vi "Check_UI2R_Validity.vi"(8 "error in (no error)":errorcluster, 9 "ControlValueUpdates[] in":T1[](array[typedef]), 10 "UI Filepath in":path, 11 "UI_Interaction_Manager in":refnum<class "UI_Interaction_Manager.lvclass">) -> (0 "error out":errorcluster, 1 "ControlValueUpdates[] out":T1[](array[typedef]), 2 "Valid?":bool, 3 "UI_Interaction_Manager out":refnum<class "UI_Interaction_Manager.lvclass">)   [LabVIEW 2011, in "UI_Interaction_Manager.lvclass"]
uses:
  UI_Interaction_Manager.lvclass
  TypeDefs/ControlValueUpdate.ctl
  UI_Interaction_Manager.lvclass/UI_Interaction_Manager.ctl
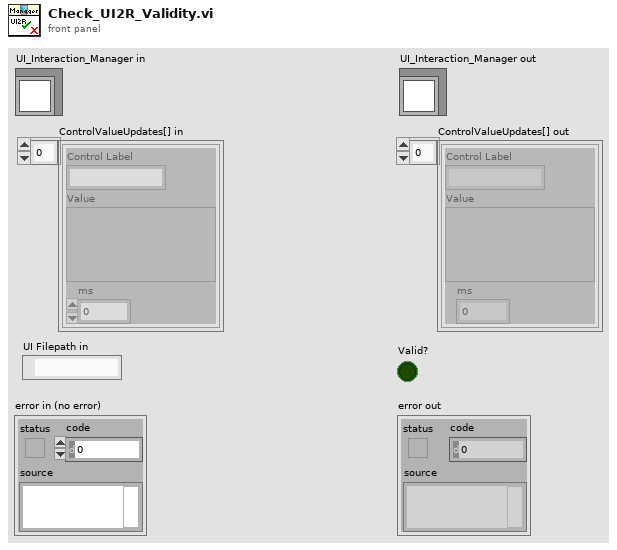
[diagram p1: front panel]
types:
  T1 = typedef "UI_Interaction_Manager.lvclass/ControlValueUpdate.ctl" = cluster{"Control Label":string, "Value":variant, "ms":u32}
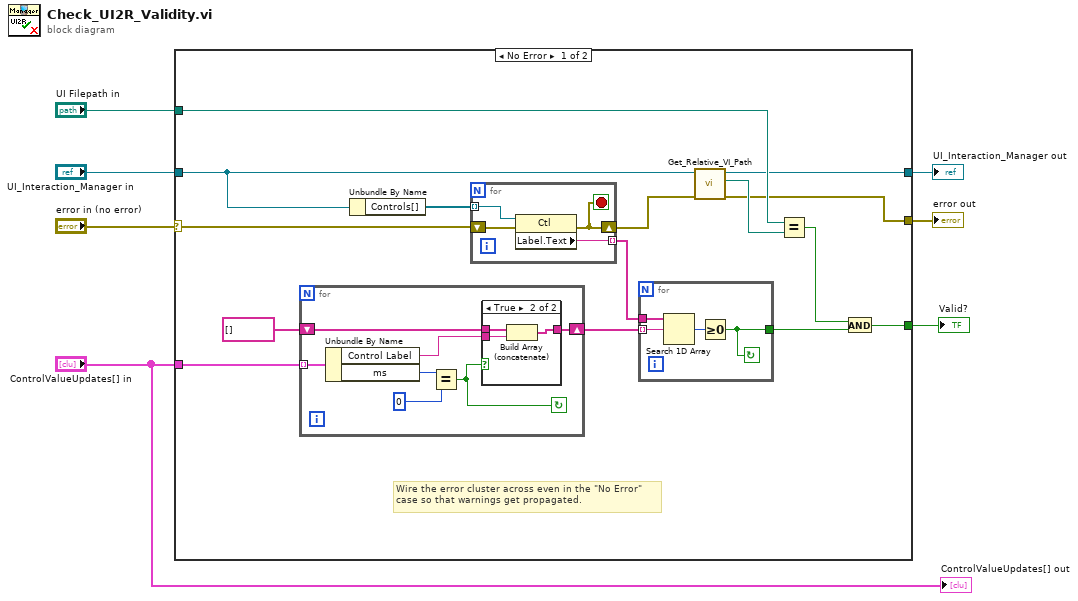
[diagram p0: block diagram]
diagram:
  n1 = case shown="No Error" "error in (no error)" {
    selector: "error in (no error)" -> [w16 w43]
    tunnel: [w11 w43] -> w6
    tunnel: [w12 w42] -> w4
    tunnel: "UI_Interaction_Manager in" -> [w17 w42]
    tunnel: "UI Filepath in" -> [w14 _]
    tunnel: "ControlValueUpdates[] in" -> [w22 _]
    tunnel: [w8 _] -> w1
    frame No Error {
      # "Wire the error cluster across even in the \"No Error\"\ncase so that warnings get propagated."
      n2 = for {
        tunnel: w22 -> [w37] mode=indexing
        shift-right: [w31] -> w19
        shift-left: string[] [] -> [w34]
        stop <- w33 continue-if-true
        n3 = Unbundle By Name(w37) -> ("Control Label"=w32:string, "ms"=w36:u32)
        n4 = Equal?(x=w36, y=u32 0) -> (x = y?=w33:bool)
        n5 = case shown="True" w33 {
          tunnel: w34 -> [w38 w41]
          tunnel: w32 -> [_ w40]
          tunnel: [w38 w39] -> w31
          frame False {
          }
          frame True {
            n6 = Build Array (concatenate)(w41, w40) -> (w39:string[])
          }
        }
      }
      n7 = Unbundle By Name(w17) -> ("Controls[]"=w20:refnum<vi>[])
      n8 = for {
        tunnel: w20 -> [w27] mode=indexing
        tunnel: [w30] -> w18 mode=indexing
        shift-right: [w28] -> w15
        shift-left: w16 -> [w29]
        stop <- w28 stop-if-true
        n9 = property class="Ctl"(reference=w27, error in=w29) -> (error out=w28:errorcluster, "Label.Text"=w30:string)  [unwired: 1 out]
      }
      n10 = for {
        tunnel: w19 -> [w26] mode=indexing
        tunnel: w18 -> [w25]
        tunnel: [w23] -> w10
        stop <- w23 continue-if-true
        n11 = Search 1D Array(1D array=w25, element=w26) -> (index of element=w24:i32)  [unwired: 1 in]
        n12 = Greater Or Equal To 0?(x=w24) -> (x >= 0?=w23:bool)
      }
      n13 = call "Get_Relative_VI_Path.vi"("error in (no error)"=w15, "UI_Interaction_Manager in"=w17) -> ("error out"=w11:errorcluster, "Relative VI Path"=w13:path, "UI_Interaction_Manager out"=w12:refnum<class "UI_Interaction_Manager.lvclass">)  [unwired: 7 in]
      n14 = Equal?(x=w14, y=w13) -> (x = y?=w9:bool)
      n15 = And(x=w9, y=w10) -> (x .and. y?=w8:bool)
    }
    frame Error {
    }
  }
  "error out" <- w6
  "UI_Interaction_Manager out" <- w4
  "Valid?" <- w1
  "ControlValueUpdates[] out" <- "ControlValueUpdates[] in"
